vi "SaveOffsets.vi"(2 "error in":errorcluster, 4 "configuration file path":path) -> (0 "error out":errorcluster)   [LabVIEW 2014]
uses:
  <vilib>/Utility/config.llb/Write Key (Double).vi
  Robot Global Data.vi
  <vilib>/Utility/config.llb/NI_LVConfig.lvlib
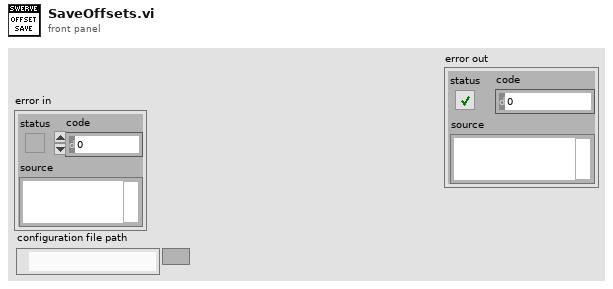
[diagram p1: front panel]
types:
  T1 = typedef "WPI_MotorControlDeviceRef.ctl" = cluster{"DeviceStatus":errorcluster, "Type":T2, "PWM":cluster{"Controller":T3, "PWM Channel":T4, "DeadBand":T5}, "CAN":cluster{"Device Number":u8, "Control Mode":T6, "Semaphore":T7, "Max Vout":dbl, "TalonSRX Control Mode":T8}, "Invert":bool, "TransformRef":T9, "InvTransformRef":T9}
  T2 = typedef "WPI_MotorControlType.ctl" = enum16{"PWM", "CAN", "CANTalonSRX"}
  T3 = typedef "FPGA_TypedefDigitalModule.ctl" = enum16{"Controller 1"}
  T4 = typedef "FPGA_DIOPWMChannel.ctl" = enum8{"PWM 0", "PWM 1", "PWM 2", "PWM 3", "PWM 4", "PWM 5", "PWM 6", "PWM 7", "PWM 8", "PWM 9", "PWM MXP 0", "PWM MXP 1", "PWM MXP 2", "PWM MXP 3", "PWM MXP 4", "PWM MXP 5", "PWM MXP 6", "PWM MXP 7", "PWM MXP 8", "PWM MXP 9", "Invalid"}
  T5 = typedef "WPI_PWMDeadband.ctl" = cluster{"Name":string, "maxPositivePwm":i32, "minPositivePwm":i32, "centerPwm":i32, "maxNegativePwm":i32, "minNegativePwm":i32, "angularRange":u16}
  T6 = typedef "WPI_CANJaguar_ControlMode.ctl" = enum8{"Percent VBus", "Current", "Speed", "Position", "Voltage"}
  T7 = typedef "Semaphore RefNum" = refnum<k1>
  T8 = typedef "WPI_CANTalonSRX_APIControlMode.ctl" = enum8{"Percent VBus", "Speed", "Position", "Slave", "Unchanged / Invalid"}
  T9 = typedef "WPI_PWMTransform_ConPane.ctl" = refnum<vi>
  T10 = cluster{"FL Steering":T1, "FR Steering":T1, "RL Steering":T1, "RR Steering":T1}
  T11 = typedef "WPI_CANTalonSRX_GlobalStatus.ctl" = cluster{"Applied Throttle":dbl, "Module Enabled":bool, "CAN Error":errorcluster, "Closed Loop Error":dbl, "Forward Limit Switch Closed":bool, "Reverse Limit Switch Closed":bool, "Sensor Position":dbl, "Sensor Velocity":dbl, "Current":dbl, "Sticky Fault - Over Temp":bool, "Sticky Fault - Under Voltage":bool, "Sticky Fault - Forward Limit":bool, "Sticky Fault - Reverse Limit":bool, "Sticky Fault - Forward Soft Limit":bool, "Sticky Fault - Reverse Soft Limit":bool, "Brake is Enabled":bool, "Encoder Position":dbl, "Encoder Velocity":dbl, "Encoder Index Count":dbl, "Encoder A Pin State":bool, "Encoder B Pin State":bool, "Encoder Index Pin State":bool, "Analog In":dbl, "Analog In Velocity":dbl, "Temperature (C)":dbl, "Battery Voltage":dbl}
  T12 = typedef "NI_LVConfig.lvlib/Config Data RefNum.ctl" = refnum<k1>
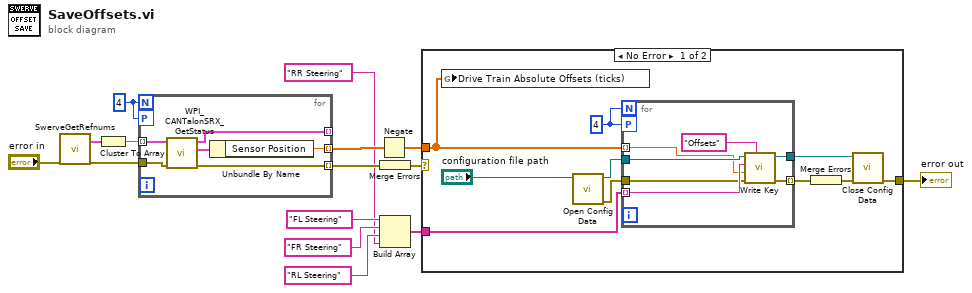
[diagram p0: block diagram]
diagram:
  w13 = 4
  n1 = call "SwerveGetRefnums.vi"("error in (no error)"="error in") -> ("Steering"=w11:T10, "error out"=w12:errorcluster)  [unwired: 8 in, 9 out]
  n2 = Cluster To Array(cluster=w11) -> (array=w10:T1[])
  n3 = for {
    N: w13 -> [_]
    tunnel: [w21] -> w8 mode=indexing
    tunnel: [w17] -> _ mode=indexing
    tunnel: w12 -> [w19]
    tunnel: [w18] -> w9 mode=indexing
    workers-P: w13 -> [_]
    tunnel: w10 -> [w16] mode=indexing
    n4 = call <vilib>:"WPI_CANTalonSRX_GetStatus.vi"("error in (no error)"=w19, "CAN Talon SRX Ref"=w16) -> ("error out"=w18:errorcluster, "Talon SRX Status"=w20:T11, "CAN Talon SRX Ref Out"=w17:T1)  [unwired: 7 in]
    n5 = Unbundle By Name(w20) -> ("Sensor Position"=w21:dbl)
  }
  n6 = Negate(x=w8) -> (-x=w7:dbl[])
  n7 = Merge Errors(w9) -> (w15:errorcluster)
  n8 = Build Array("FL Steering", "FR Steering" ("element"), "RL Steering" ("element"), "RR Steering" ("element")) -> (w2:string[])
  n9 = case shown="No Error" w15 {
    selector: w15 -> [_ w39]
    tunnel: w7 -> [w29 _]
    tunnel: w2 -> [w30 _]
    tunnel: [w22 w39] -> w1
    frame No Error {
      w31 = 4
      n10 = global write "Robot Global Data.vi" "Drive Train Absolute Offsets (ticks)"(w29) -> ()
      n11 = call <vilib>:"Open Config Data.vi"("configuration file path"="configuration file path") -> ("error out"=w25:errorcluster, "refnum"=w27:T12)  [unwired: 2 in, 7 out]
      n12 = for {
        N: w31 -> [_]
        tunnel: w27 -> [w38]
        workers-P: w31 -> [_]
        tunnel: w30 -> [w37] mode=indexing
        tunnel: w29 -> [w36] mode=indexing
        tunnel: [w35] -> w28 mode=indexing
        tunnel: w25 -> [w33]
        tunnel: [w32] -> w23
        n13 = call-poly <vilib>:"Write Key.vi"("section"="Offsets", "error in (no error)"=w33, "value"=w36, "key"=w37, "refnum"=w38) -> ("error out"=w35:errorcluster, "refnum out"=w32:T12)  [unwired: 3 in, 2 out]
      }
      n14 = Merge Errors(w28) -> (w24:errorcluster)
      n15 = call <vilib>:"Close Config Data.vi"("error in (no error)"=w24, "refnum"=w23) -> ("error out"=w22:errorcluster)  [unwired: 8 in, 1 out]
    }
    frame Error {
    }
  }
  "error out" <- w1
